vi "dbc-constructor.vi"(8 "error in (no error)":errorcluster, 9 "signal.results":refnum<vi>, 10 "table.ref in":refnum<vi>, 11 "tree.ref.in":refnum<vi>) -> (0 "error out":errorcluster, 3 "dbc out":refnum<class "dbc.lvclass">)   [LabVIEW 2015, in "dbc.lvclass"]
uses:
  dbc.lvclass
  class.can.table/CAN_table.ctl
  controls/dbc-file-data.ctl
  controls/dbc-content-data.ctl
  controls/dbc-active-item.ctl
  dbc.lvclass/dbc.ctl
  class.bFrameIO/bFrameIO.lvclass
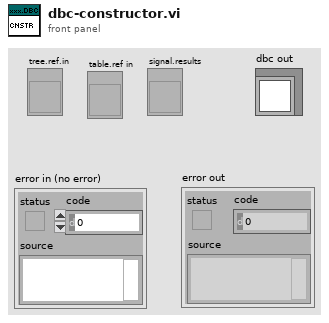
[diagram p1: front panel]
types:
  T1 = enum32{"None", "LabVIEW", "Mac OS", "Windows", "Default"}
  T2 = typedef "dbc-active-item.ctl" = cluster{"active.frame.tag":string, "activeItemTag":string, "indent.lvl":i32, "symbol":i32}
  T3 = typedef "dbc-content-data.ctl" = cluster{"Number of Clusters":i32, "Number of Frames ":i32[], "Clusters":string[], "Frames":string[][], "Signals":string[][][], "Number of Signals":i32[][]}
  T4 = typedef "dbc-file-data.ctl" = cluster{"dbc.ref":refnum<k21>, "dbc.file":path, "alias":string}
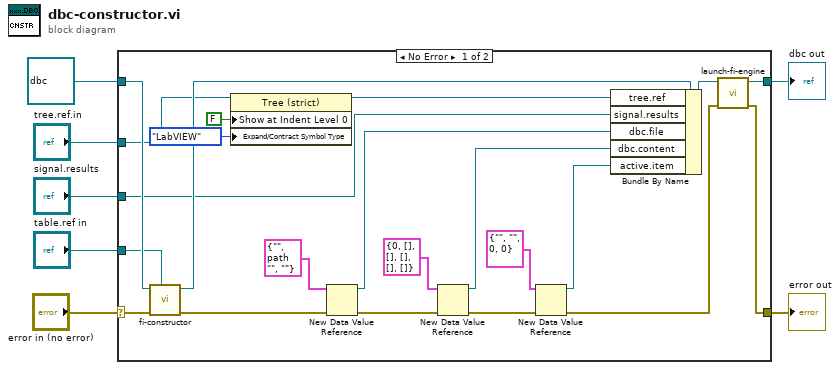
[diagram p0: block diagram]
diagram:
  n1 = case shown="No Error" "error in (no error)" {
    selector: "error in (no error)" -> [w28 w31]
    tunnel: [w18 w31] -> w6
    tunnel: [w19 w30] -> w4
    tunnel: refnum<class "dbc.lvclass"> refnum ("dbc in") -> [w21 w30]
    tunnel: "tree.ref.in" -> [w16 _]
    tunnel: "table.ref in" -> [w15 _]
    tunnel: "signal.results" -> [w14 _]
    frame No Error {
      n2 = call "fi-constructor.vi"("table.ref in"=w15, "error in (no error)"=w28, "frameInput in"=w21) -> ("error out"=w22:errorcluster, "frameInput out"=w20:refnum<class "dbc.lvclass">)  [unwired: 7 in]
      n3 = property class="Tree (strict)"(reference=w16, "Show at Indent Level 0"=FALSE ("Expand/Contract Symbol:Show Symbol at Root"), "Expand/Contract Symbol Type"=T1."LabVIEW" ("Expand/Contract Symbol:Symbol Type")) -> (reference out=w10:refnum<vi>)  [unwired: 1 in, 1 out]
      n4 = New Data Value Reference(data value=T4 {"dbc.ref"="", "dbc.file"=path "", "alias"=""} ("dbc.file"), error in=w22) -> (data value reference=w24:refnum<data-value>, error out=w29:errorcluster)
      n5 = New Data Value Reference(data value=T3 {"Number of Clusters"=0, "Number of Frames "=[], "Clusters"=[], "Frames"=[], "Signals"=[], "Number of Signals"=[]} ("Cluster"), error in=w29) -> (data value reference=w23:refnum<data-value>, error out=w17:errorcluster)
      n6 = New Data Value Reference(data value=T2 {"active.frame.tag"="", "activeItemTag"="", "indent.lvl"=0, "symbol"=0} ("active.item"), error in=w17) -> (data value reference=w11:refnum<data-value>, error out=w13:errorcluster)
      n7 = Bundle By Name(cluster=w20, "tree.ref"=w10, "signal.results"=w14, "dbc.file"=w24, "dbc.content"=w23, "active.item"=w11) -> (w25:refnum<class "dbc.lvclass">)
      n8 = call "launch-fi-engine.vi"("error in (no error)"=w13, "fi in"=w25) -> ("error out"=w18:errorcluster, "fi out"=w19:refnum<class "dbc.lvclass">)  [unwired: 8 in]
    }
    frame Error {
    }
  }
  "error out" <- w6
  "dbc out" <- w4
